vi "Configure Channels.vi"(8 "error in":errorcluster, 11 "AI DAQmx CFG in":refnum<class "AI Current DAQmx Cont CFG.lvclass">) -> (0 "error out":errorcluster, 3 "AI DAQmx CFG out":refnum<class "AI Current DAQmx Cont CFG.lvclass">)   [LabVIEW 2023, in "AI Current DAQmx Cont CFG.lvclass"]
uses:
  AI Current DAQmx Cont CFG.lvclass
  DAQmx/DAQmx BufferLastReadsDBL/DAQmx BufferLastReadsDBL.lvclass/DAQmx BufferLastReadsDBL.ctl
  DAQmx/DAQmx Base CFG/DAQmx Base CFG.lvclass/DAQmx Base CFG.ctl
  Configuration/Configuration JSON/Configuration JSON Base/CFG JSON.lvclass/CFG JSON.ctl
  be60a397-d282-4f5e-a878-4098099e3210.vi
  be60a397-d282-4f5e-a878-4098099e3210.vi/a4169a97-72fc-4003-a778-603cf20cafa0.vi
  <vilib>/JDP Science/JSONtext/Find Item.vi
  <vilib>/JDP Science/JSONtext/Next JSON Value.vi
  <vilib>/JDP Science/JSONtext/String Subset.vi
  <vilib>/JDP Science/JSONtext/Parsing/Advance past next JSON Value (inlined COPY).vi
  <vilib>/JDP Science/JSONtext/Parsing/Advance past whitespace.vi
  <vilib>/JDP Science/JSONtext/Parsing/Advance past String.vi
  <vilib>/JDP Science/JSONtext/Parsing/Advance past Number.vi
  <vilib>/JDP Science/JSONtext/Parsing/Advance past Line Ending.vi
  <vilib>/JDP Science/JSONtext/Parsing/Parse Full Path or Item Name.vi
  <vilib>/JDP Science/JSONtext/Parsing/Advance past Array.vi
  <vilib>/JDP Science/JSONtext/Parsing/Advance past Object.vi
  <vilib>/JDP Science/JSONtext/support/Error Cluster From Code.vi
  <vilib>/JDP Science/JSONtext/Offset/Find Item Locations by Path.vi
  <vilib>/JDP Science/JSONtext/JSON text to Variant.vi
  <vilib>/Utility/error.llb/Error Cluster From Error Code.vi
  <vilib>/JDP Science/JSONtext/LVClass Serializer/JSONtext LVClass Serializer.lvclass
  AI Current DAQmx Cont CFG.lvclass/AI Current DAQmx Cont CFG.ctl
  <vilib>/DAQmx/create/channels.llb/DAQmx Create Channel (AI-Current-Basic).vi
  Configuration/Configuration JSON/Configuration JSON Base/CFG JSON.lvclass
  DAQmx/DAQmx Base CFG/DAQmx Base CFG.lvclass
  DAQmx/DAQmx BufferLastReadsDBL/DAQmx BufferLastReadsDBL.lvclass
  DAQmx/BufferLastReadingsDBL/BufferLastReadsDBL.lvclass
  D:/git/HAL/HAL GOOP4/DAQmx/DAQmx BufferLastReadsDBL/DAQmx BufferLastReadsDBL.lvclass
  D:/git/HAL/HAL GOOP4/DAQmx/DAQmx Base CFG/DAQmx Base CFG.lvclass
  D:/git/HAL/HAL GOOP4/CFG Target/CFG Target.lvclass
  D:/git/HAL/HAL GOOP4/Configuration/Configuration Semaphore/CFG Semaphore.lvclass
  D:/git/HAL/HAL GOOP4/Configuration/Configuration JSON/Configuration JSON Base/CFG JSON.lvclass
  D:/git/HAL/HAL GOOP4/Interfaces/IConfigure/IConfigure.lvclass
  D:/git/HAL/HAL GOOP4/AI/AI Current DAQmx Cont CFG/AI Current DAQmx Cont CFG.lvclass
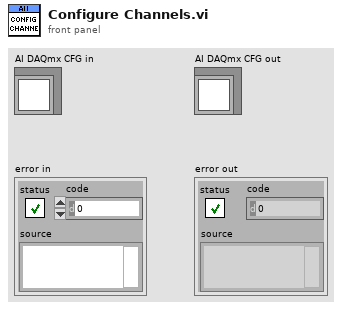
[diagram p1: front panel]
types:
  T1 = cluster{"Name":string, "Enabled":bool, "Max Value":dbl, "Min Value":dbl, "Input Terminal CFG":string, "Units":string, "Shunt Resistor Location":string, "External Shunt Resistor Value":dbl}[]
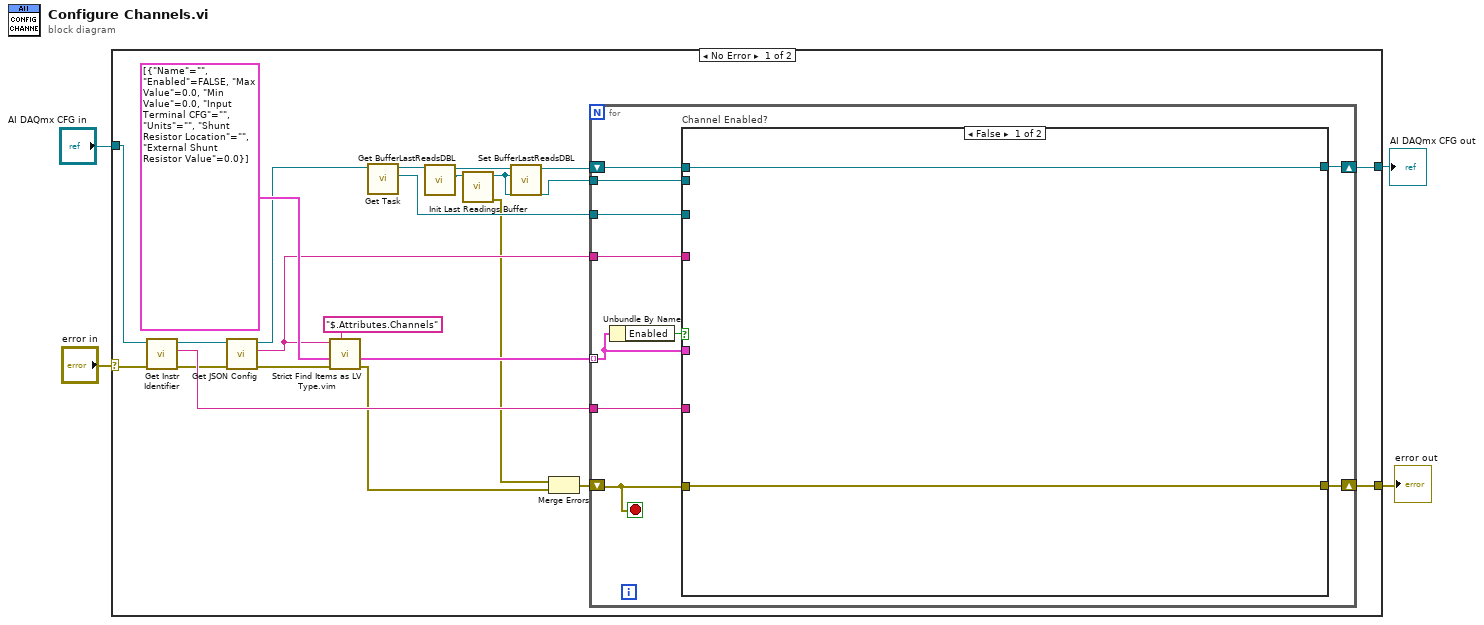
[diagram p0: block diagram]
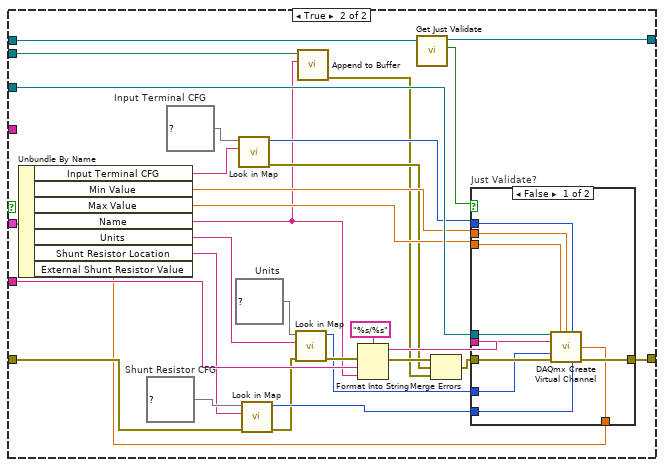
[diagram p2: hidden frame]
diagram:
  n1 = case shown="No Error" "error in" {
    selector: "error in" -> [w20 w79]
    tunnel: "AI DAQmx CFG in" -> [w17 w80]
    tunnel: [w21 w79] -> w2
    tunnel: [w7 w80] -> w1
    frame No Error {
      n2 = call-dynamic "Get Instr Identifier.vi"("error in"=w20, "Configuration Base in"=w17) -> ("error out"=w16:errorcluster, "Instr Ident"=w22:string, "Configuration Base out"=w23:refnum<class "AI Current DAQmx Cont CFG.lvclass">)  [unwired: 7 in]
      n3 = call "Get JSON Config.vi"("CFG Base in"=w23) -> ("<JSON>Config>"=w19:string, "CFG Base out"=w15:refnum<class "AI Current DAQmx Cont CFG.lvclass">)  [unwired: 9 in]
      n4 = call "Strict Find Items as LV Type.vim"("$Path or Item Name"="$.Attributes.Channels", "error in"=w16, "Data Type and Default Value"=T1 [{"Name"="", "Enabled"=FALSE, "Max Value"=0.0, "Min Value"=0.0, "Input Terminal CFG"="", "Units"="", "Shunt Resistor Location"="", "External Shunt Resistor Value"=0.0}], "JSON"=w19) -> ("error out"=w8:errorcluster, "Data out"=w18:T1)  [unwired: 6 in]
      n5 = call "Get Task.vi"("DAQmx Base CFG in"=w15) -> ("Task"=w13:refnum<k21>, "DAQmx Base CFG out"=w12:refnum<class "AI Current DAQmx Cont CFG.lvclass">)  [unwired: 9 in]
      n6 = call "Get BufferLastReadsDBL.vi"("DAQmx BufferLastReadsDBL in"=w12) -> ("BufferLastReadsDBL.lvclass"=w11:refnum<class "BufferLastReadsDBL.lvclass">, "DAQmx BufferLastReadsDBL out"=w10:refnum<class "AI Current DAQmx Cont CFG.lvclass">)  [unwired: 9 in]
      n7 = call "Init Last Readings Buffer.vi"("BufferLastReadingsDBL in"=w11) -> ("error out"=w9:errorcluster, "BufferLastReadingsDBL out"=w5:refnum<class "BufferLastReadsDBL.lvclass">)  [unwired: 9 in]
      n8 = call "Set BufferLastReadsDBL.vi"("BufferLastReadsDBL.lvclass"=w5, "DAQmx BufferLastReadsDBL in"=w10) -> ("DAQmx BufferLastReadsDBL out"=w6:refnum<class "AI Current DAQmx Cont CFG.lvclass">)  [unwired: 9 in]
      n9 = Merge Errors(w9, w8) -> (w14:errorcluster)
      n10 = for {
        tunnel: w18 -> [w32] mode=indexing
        shift-right: [w35] -> w21
        shift-left: w14 -> [w34]
        tunnel: w22 -> [w33]
        tunnel: w19 -> [w31]
        tunnel: w13 -> [w30]
        shift-right: [w29] -> w7
        shift-left: w6 -> [w28]
        tunnel: w5 -> [w26]
        stop <- w34 stop-if-true
        n11 = Unbundle By Name(w32) -> ("Enabled"=w27:bool)
        n12 = case "Channel Enabled?" shown="False" w27 {
          tunnel: [w37 w66] -> w35
          tunnel: w34 -> [w37 w44]
          tunnel: w33 -> [_ w60]
          tunnel: w32 -> [_ w67]
          tunnel: [w36 w63] -> w29
          tunnel: w31 -> [_ _]
          tunnel: w30 -> [_ w65]
          tunnel: w28 -> [w36 w64]
          tunnel: w26 -> [_ w40]
          frame False {
          }
          frame True {
            w48 = map{string, i32} {"External"=10167, "Internal"=10200, "default"=-1}  # Shunt Resistor CFG
            w54 = map{string, i32} {"Amps"=10342, "From Custom Scale"=10065}  # Units
            w56 = map{string, i32} {"Differential"=10106, "NRSE"=10078, "Pseudodifferential"=12529, "RSE"=10083, "default"=-1}  # Input Terminal CFG
            n13 = Unbundle By Name(w67) -> ("Input Terminal CFG"=w55:string, "Min Value"=w52:dbl, "Max Value"=w51:dbl, "Name"=w39:string, "Units"=w49:string, "Shunt Resistor Location"=w41:string, "External Shunt Resistor Value"=w42:dbl)
            n14 = call "Look in Map.vi"("Key"=w55, "Map"=w56) -> ("error out"=w47:errorcluster, "Value"=w53:i32)  [unwired: 8 in]
            n15 = call "Look in Map.vi"("error in"=w44, "Key"=w41, "Map"=w48) -> ("error out"=w43:errorcluster, "Value"=w45:i32)  [unwired: 7 in]
            n16 = call "Look in Map.vi"("error in"=w43, "Key"=w49, "Map"=w54) -> ("error out"=w50:errorcluster, "Value"=w46:i32)  [unwired: 7 in]
            n17 = call "Append to Buffer.vi"("Channel"=w39, "BufferLastReadingsDBL in"=w40) -> ("error out"=w38:errorcluster)  [unwired: 8 in, 1 out]
            n18 = Format Into String(format string="%s/%s", error in=w50, w60, w39) -> (resulting string=w58:string, error out=w59:errorcluster)  [unwired: 1 in]
            n19 = call "Get Just Validate.vi"("CFG JSON Base in"=w64) -> ("Just Validate"=w62:bool, "CFG JSON Base out"=w63:refnum<class "AI Current DAQmx Cont CFG.lvclass">)  [unwired: 9 in]
            n20 = Merge Errors(w59, w47, w38) -> (w57:errorcluster)
            n21 = case "Just Validate?" shown="False" w62 {
              tunnel: w57 -> [w77 w78]
              tunnel: w58 -> [w74 _]
              tunnel: w65 -> [w76 _]
              tunnel: [w75 w78] -> w66
              tunnel: w53 -> [w73 _]
              tunnel: w52 -> [w72 _]
              tunnel: w51 -> [w71 _]
              tunnel: w46 -> [w70 _]
              tunnel: w45 -> [w69 _]
              tunnel: w42 -> [w68 _]
              frame False {
                n22 = call-poly <vilib>:"DAQmx Create Virtual Channel.vi"("task in"=w76, "maximum value"=w71, "minimum value"=w72, "input terminal configuration"=w73, "physical channels"=w74, "external shunt resistor value"=w68, "units"=w70, "error in"=w77, "shunt resistor location"=w69) -> ("error out"=w75:errorcluster)  [unwired: 5 in, 1 out]
              }
              frame True {
              }
            }
          }
        }
      }
    }
    frame Error {
    }
  }
  "error out" <- w2
  "AI DAQmx CFG out" <- w1
